vi "Delete Scale Wrapper.vi"(8 "error in (no error)":errorcluster, 10 "index":i32, 11 "Scaling configuration in":refnum<class "Scaling configuration.lvclass">) -> (0 "error out":errorcluster, 2 "Deleted Scale":T2, 3 "Scaling configuration out":refnum<class "Scaling configuration.lvclass">)   [LabVIEW 2014, in "Scaling configuration.lvclass"]
uses:
  Scaling configuration.lvclass
  <vilib>/NI/Tag Bus Module Framework/channel/TBM channel.lvclass
  controls/scale data types.ctl
  Scaling configuration.lvclass/Scaling configuration.ctl
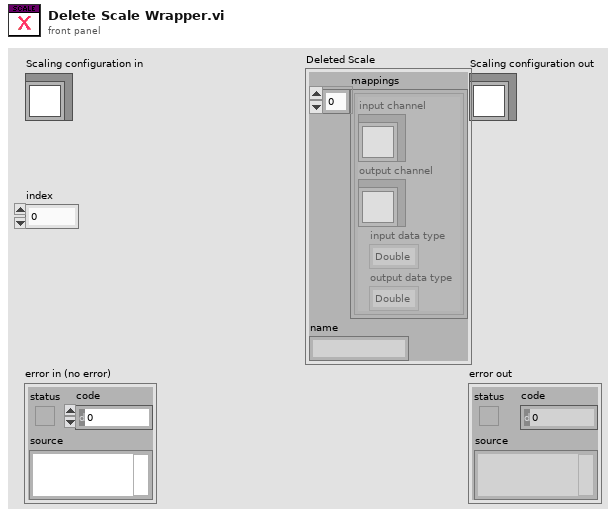
[diagram p1: front panel]
types:
  T1 = typedef "Scaling configuration.lvclass/scale data types.ctl" = enum16{"Double", "Single", "I64", "I32", "I16", "I8", "U64", "U32", "U16", "U8", "Boolean"}
  T2 = cluster{"mappings":cluster{"input channel":refnum<class "TBM channel.lvclass">, "output channel":refnum<class "TBM channel.lvclass">, "input data type":T1, "output data type":T1}[], "name":string}
  T3 = cluster{"mappings":cluster{"input channel":refnum<class "TBM channel.lvclass">, "output channel":refnum<class "TBM channel.lvclass">, "input data type":T1, "output data type":T1}[], "name":string}[]
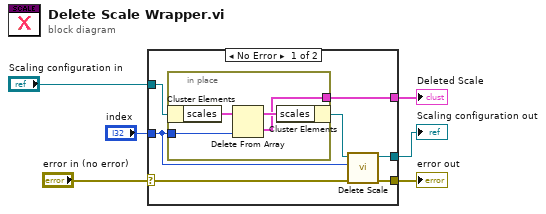
[diagram p0: block diagram]
diagram:
  n1 = case shown="No Error" "error in (no error)" {
    selector: "error in (no error)" -> [w9 w19]
    tunnel: [w8 w19] -> w5
    tunnel: [w7 w18] -> w3
    tunnel: "Scaling configuration in" -> [w13 w18]
    tunnel: "index" -> [w10 _]
    tunnel: [w12 _] -> w1
    frame No Error {
      n2 = in-place {
        in-place-border: w10 -> [w16]
        in-place-border: [w14] -> w12
        n3 = in-place-cluster #1(w13) -> ("scales"=w17:T3)
        n4 = Delete From Array(array=w17, index=w16) -> (deleted portion=w14:T2, array with subset deleted=w15:T3)  [unwired: 1 in]
        n5 = in-place-cluster #1("scales"=w15) -> (w11:refnum<class "Scaling configuration.lvclass">)
      }
      n6 = call-dynamic "Delete Scale.vi"("error in (no error)"=w9, "index"=w10, "Scaling configuration in"=w11) -> ("error out"=w8:errorcluster, "Scaling configuration out"=w7:refnum<class "Scaling configuration.lvclass">)  [unwired: 7 in]
    }
    frame Error {
    }
  }
  "error out" <- w5
  "Scaling configuration out" <- w3
  "Deleted Scale" <- w1
